vi "CoboltLaser_ComPortOpen.vi"(0 "ComPort":refnum<visa-resource-name>, 5 "error in (no error)":errorcluster) -> (14 "ComPort Out":refnum<visa-resource-name>, 19 "error out":errorcluster)   [LabVIEW 2012, in "Cobolt.lvclass"]
doc: "Use this template to build a VI to use as a subVI."
uses:
  Template/Cobolt.lvclass
  <vilib>/Instr/_visa.llb/VISA Configure Serial Port (Instr).vi
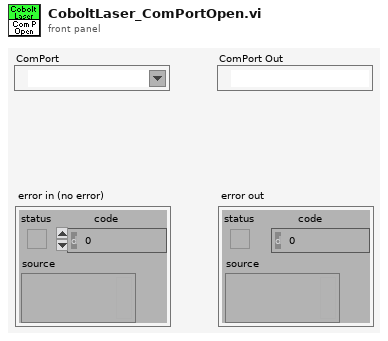
[diagram p1: front panel]
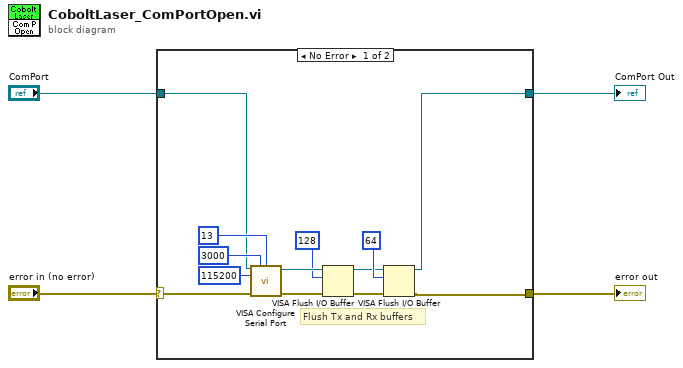
[diagram p0: block diagram]
diagram:
  n1 = case shown="No Error" "error in (no error)" {
    selector: "error in (no error)" -> [w10 w19]
    tunnel: [w11 w19] -> w3
    tunnel: "ComPort" -> [w6 w18]
    tunnel: [w5 w18] -> w1
    frame No Error {
      # "Flush Tx and Rx buffers"
      n2 = call-poly "VISA Configure Serial Port"("VISA resource name"=w6, "timeout (10sec)"=u32 3000, "termination char\n(0xA = '\\n' = LF)"=u8 13 ("termination char\n(0xA = '\\n' = LF)"), "baud rate (9600)"=u32 115200, "error in (no error)"=w10) -> ("VISA resource name out"=w17:refnum<visa-resource-name>, "error out"=w16:errorcluster)  [unwired: 4 in, 5 out]
      n3 = VISA Flush I/O Buffer(VISA resource name=w17, mask (16)=u16 128, error in (no error)=w16) -> (VISA resource name out=w13:refnum<visa-resource-name>, error out=w12:errorcluster)
      n4 = VISA Flush I/O Buffer(VISA resource name=w13, mask (16)=u16 64, error in (no error)=w12) -> (VISA resource name out=w5:refnum<visa-resource-name>, error out=w11:errorcluster)
    }
    frame Error {
    }
  }
  "error out" <- w3
  "ComPort Out" <- w1
